vi "Begin.vi"(8 "error in":errorcluster) -> (0 "error out":errorcluster)   [LabVIEW 2016]
doc: "Called before other user functions, this VI is expected to open initial I/O refnums, load in file data, and do all program initialization. Notice that the <B>error out</B> terminal is simply used for data flow. Wiring it to other structures or subVIs ensures that this VI runs first."
uses:
  <vilib>/Rock Robotics/SystemInterfaces/DIO/FPGA_DIOPWMChannel.ctl
  <vilib>/Rock Robotics/WPI/SafetyOutput/WPI_SafetyOutputConfigMenu.ctl
  <vilib>/Rock Robotics/WPI/DriverStation/WPI_DriverStationRobotMode2.ctl
  <vilib>/Rock Robotics/WPI/Joystick/WPI_JoystickDeviceEnum.ctl
  <vilib>/Rock Robotics/WPI/Solenoid/WPI_SolenoidChannel.ctl
  <vilib>/Rock Robotics/SystemInterfaces/DIO/FPGA_DIOChannel.ctl
  <vilib>/Rock Robotics/WPI/Encoder/WPI_EncoderType.ctl
  <vilib>/Rock Robotics/WPI/RobotDrive/WPI_RobotDriveOpen2MotorWithTalon.vi
  Robot Global Data.vi
  <vilib>/Rock Robotics/Network Tables/SD Write String Array.vi
  <vilib>/Rock Robotics/WPI/Utilities/WPI_GetSetVariantRefNum.vi
  <vilib>/Rock Robotics/WPI/Solenoid/WPI_SolenoidOpenSingle.vi
  <vilib>/Rock Robotics/WPI/Counter/WPI_CounterDigitalInputToDigitalSource.vi
  <vilib>/Rock Robotics/WPI/MotorControl/WPI_MotorControlOpen VictorSP.vi
  <vilib>/Rock Robotics/WPI/Ultrasonic/WPI_SonarSRF04DigitalOpen.vi
  <vilib>/Rock Robotics/WPI/Ultrasonic/WPI_SonarSRF04DigitalRefNum Registry Set.vi
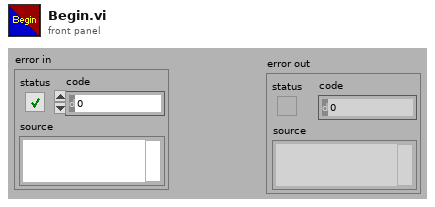
[diagram p1: front panel]
types:
  T1 = typedef "FPGA_DIOChannel.ctl" = enum8{"DIO 0", "DIO 1", "DIO 2", "DIO 3", "DIO 4", "DIO 5", "DIO 6", "DIO 7", "DIO 8", "DIO 9", "DIO MXP 0", "DIO MXP 1", "DIO MXP 2", "DIO MXP 3", "DIO MXP 4", "DIO MXP 5", "DIO MXP 6", "DIO MXP 7", "DIO MXP 8", "DIO MXP 9", "DIO MXP 10", "DIO MXP 11", "DIO MXP 12", "DIO MXP 13", "DIO MXP 14", "DIO MXP 15", "SPI Port CS1", "SPI Port CS2", "SPI Port CS3", "SPI Port MISO", "SPI Port MOSI", "Invalid"}
  T2 = typedef "FPGA_DIOPWMChannel.ctl" = enum8{"PWM 0", "PWM 1", "PWM 2", "PWM 3", "PWM 4", "PWM 5", "PWM 6", "PWM 7", "PWM 8", "PWM 9", "PWM MXP 0", "PWM MXP 1", "PWM MXP 2", "PWM MXP 3", "PWM MXP 4", "PWM MXP 5", "PWM MXP 6", "PWM MXP 7", "PWM MXP 8", "PWM MXP 9", "Invalid"}
  T3 = typedef "WPI_EncoderType.ctl" = enum16{"1x", "2x", "4x"}
  T4 = typedef "WPI_SolenoidChannel.ctl" = enum8{"Solenoid 0", "Solenoid 1", "Solenoid 2", "Solenoid 3", "Solenoid 4", "Solenoid 5", "Solenoid 6", "Solenoid 7", "Invalid"}
  T5 = typedef "WPI_JoystickDeviceEnum.ctl" = enum16{"USB 0", "USB 1", "USB 2", "USB 3", "USB 4", "USB 5"}
  T6 = typedef "WPI_DriverStationRobotMode2.ctl" = enum16{"Autonomous Disabled", "Autonomous Enabled", "Teleop Disabled", "Teleop Enabled", "Disconnected", "Finish", "Test Disabled", "Test Enabled", "Emergency Stopped"}
  T7 = typedef "WPI_SafetyOutputConfigMenu.ctl" = enum16{"Enable", "Disable"}
  T8 = typedef "WPI_DigitalInputDevRef.ctl" = cluster{"DevStatus":errorcluster, "DIO Channel":T1}
  T9 = typedef "FPGA_CounterEncoderSourceConvertionLVSourceType.ctl" = cluster{"DevStatus":errorcluster, "AnalogTriggerMode?":bool, "DigitalMode":cluster{"DIO Channel":T10}, "AnalogTriggerMode":cluster{"AnalogTriggerIndex":T11, "OutputType":T12}}
  T10 = typedef "FPGA_DIODigitalSourceChannel.ctl" = enum8{"DIO 0", "DIO 1", "DIO 2", "DIO 3", "DIO 4", "DIO 5", "DIO 6", "DIO 7", "DIO 8", "DIO 9", "DIO MXP 0", "DIO MXP 1", "DIO MXP 2", "DIO MXP 3", "DIO MXP 4", "DIO MXP 5", "DIO MXP 6", "DIO MXP 7", "DIO MXP 8", "DIO MXP 9", "DIO MXP 10", "DIO MXP 11", "DIO MXP 12", "DIO MXP 13", "DIO MXP 14", "DIO MXP 15", "Disabled"}
  T11 = typedef "FPGA_AnalogTriggerIndex.ctl" = enum8{"Trig 0", "Trig 1", "Trig 2", "Trig 3", "Trig 4", "Trig 5", "Trig 6", "Trig 7", "Invalid"}
  T12 = typedef "FPGA_AnalogTriggerOutType.ctl" = enum16{"InWindow", "TriggerState", "Rising", "Falling"}
  T13 = typedef "WPI_CompressorDevRef.ctl" = cluster{"DevStatus":errorcluster, "Pneumatics Control Module":u8}
  T14 = typedef "WPI_EncoderDevRef.ctl" = cluster{"DevStatus":errorcluster, "EncoderIndex":T15, "CounterIndex":T16, "DistancePerCount":dbl, "Decoding Type":T3}
  T15 = typedef "FPGA_EncoderIdx.ctl" = enum8{"Enc 0", "Enc 1", "Enc 2", "Enc 3", "Enc 4", "Enc 5", "Enc 6", "Enc 7", "Invalid"}
  T16 = typedef "FPGA_CounterCtrSystemIndex.ctl" = enum8{"Ctr 0", "Ctr 1", "Ctr 2", "Ctr 3", "Ctr 4", "Ctr 5", "Ctr 6", "Ctr 7", "Invalid"}
  T17 = typedef "WPI_SolenoidDevRef.ctl" = cluster{"DevStatus":errorcluster, "Pneumatics Control Module":u8, "Forward Solenoid Channel":T4, "Reverse Solenoid Channel":T4}
  T18 = typedef "WPI_JoystickDevRef.ctl" = cluster{"Device":T5}
  T19 = typedef "WPI_RobotDriveDevRef.ctl" = cluster{"DevStatus":errorcluster, "Motors[]":T20[], "Square Inputs":bool, "Max Output":dbl}
  T20 = typedef "WPI_MotorControlDeviceRef.ctl" = cluster{"DeviceStatus":errorcluster, "Type":T21, "PWM":cluster{"PWM Channel":T2, "DeadBand":T22}, "CAN":cluster{"Device Number":u8, "SetOutput VI Ref":variant, "GetOutput VI Ref":variant, "Enable VI Ref":variant, "Disable VI Ref":variant, "Data":variant}, "Invert":bool}
  T21 = typedef "WPI_MotorControlType.ctl" = enum16{"PWM", "CAN"}
  T22 = typedef "WPI_PWMDeadband.ctl" = cluster{"Name":string, "maxPositivePwm":i32, "minPositivePwm":i32, "centerPwm":i32, "maxNegativePwm":i32, "minNegativePwm":i32, "angularRange":u16}
  T23 = typedef "WPI_UltrasonicDeviceRef.ctl" = cluster{"DevStatus":errorcluster, "Ping Channel":T1, "Echo Channel":T1, "CntIndex":T16}
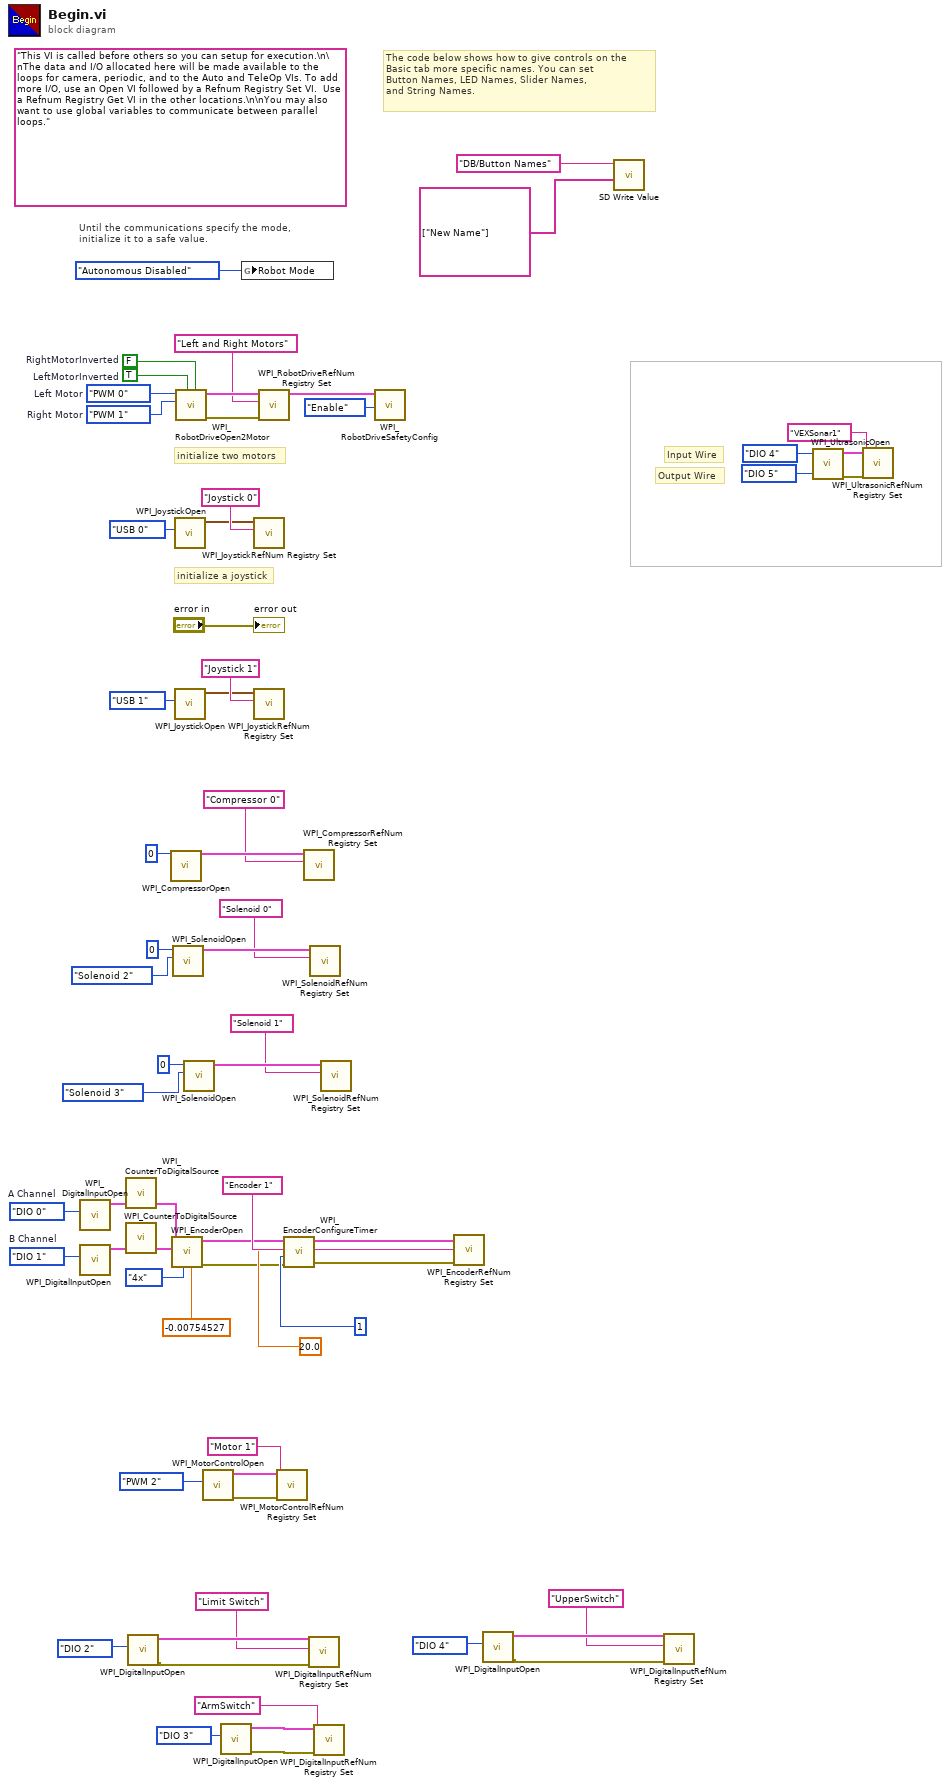
[diagram p0: block diagram]
diagram:
  w36 = FPGA_DIOChannel."DIO 1"  # B Channel
  w35 = FPGA_DIOChannel."DIO 0"  # A Channel
  (unwired) "This VI is called before others so you can setup for execution.\n\nThe data and I/O allocated here will be made available to the loops for camera, periodic, and to the Auto and TeleOp VIs. To add more I/O, use an Open VI followed by a Refnum Registry Set VI.  Use a Refnum Registry Get VI in the other locations.\n\nYou may also want to use global variables to communicate between parallel loops."
  w60 = FPGA_DIOPWMChannel."PWM 1"  # Right Motor
  w61 = FPGA_DIOPWMChannel."PWM 0"  # Left Motor
  w65 = TRUE  # LeftMotorInverted
  w66 = FALSE  # RightMotorInverted
  # "Output Wire"
  # "Input Wire"
  # "The code below shows how to give controls on the\nBasic tab more specific names. You can set\nButton Names, LED Names, Slider Names,\nand String Names."
  # "initialize a joystick"
  # "Until the communications specify the mode,\ninitialize it to a safe value."
  # "initialize two motors"
  n1 = call <vilib>:"WPI_DigitalInputOpen.vi"("DIO Channel"=w35) -> ("DigitalInputDevRef"=w32:T8)  [unwired: 1 in, 9 out]
  n2 = call <vilib>:"WPI_DigitalInputOpen.vi"("DIO Channel"=w36) -> ("DigitalInputDevRef"=w33:T8)  [unwired: 1 in, 9 out]
  n3 = call-poly <vilib>:"WPI_CounterToDigitalSource.vi"("DigitalInputDevRef"=w32) -> ("Digital Source"=w31:T9)  [unwired: 6 out]
  n4 = call-poly <vilib>:"WPI_CounterToDigitalSource.vi"("DigitalInputDevRef"=w33) -> ("Digital Source"=w34:T9)  [unwired: 6 out]
  n5 = call <vilib>:"WPI_DigitalInputOpen.vi"("DIO Channel"=FPGA_DIOChannel."DIO 2") -> ("error out"=w21:errorcluster, "DigitalInputDevRef"=w26:T8)  [unwired: 9 in]
  n6 = call <vilib>:"WPI_CompressorOpen.vi"("Pneumatics Control Module (0)"=u8 0) -> ("CompressorDevRef"=w46:T13)  [unwired: 13 in, 1 out]
  n7 = call <vilib>:"WPI_EncoderOpen.vi"("DistancePerCount"=-0.00754527, "Decoding Type"=WPI_EncoderType."4x", "BSource"=w34, "ASource"=w31) -> ("error out"=w20:errorcluster, "EncoderDevRef"=w29:T14)  [unwired: 4 in, 2 out]
  n8 = call-poly <vilib>:"WPI_SolenoidOpen.vi"("Solenoid Channel"=WPI_SolenoidChannel."Solenoid 2" ("Forward Solenoid Channel"), "Pneumatics Control Module (0)"=u8 0) -> ("SolenoidDevRef"=w44:T17)  [unwired: 8 in, 1 out]
  n9 = call <vilib>:"WPI_JoystickOpen.vi"("JoystickDevice"=WPI_JoystickDeviceEnum."USB 0") -> ("JoystickDevRef"=w55:T18)  [unwired: 10 in]
  n10 = call <vilib>:"WPI_JoystickOpen.vi"("JoystickDevice"=WPI_JoystickDeviceEnum."USB 1") -> ("JoystickDevRef"=w49:T18)  [unwired: 10 in]
  n11 = call-poly <vilib>:"WPI_RobotDriveOpen2Motor.vi"("Right Motor Inverted"=w66, "Left Motor Inverted"=w65, "Right Motor"=w60, "Left Motor"=w61) -> ("error out"=w62:errorcluster, "RobotDriveDevRef"=w64:T19)  [unwired: 1 in, 5 out]
  n12 = call-poly <vilib>:"WPI_SolenoidOpen.vi"("Solenoid Channel"=WPI_SolenoidChannel."Solenoid 3" ("Forward Solenoid Channel"), "Pneumatics Control Module (0)"=u8 0) -> ("SolenoidDevRef"=w40:T17)  [unwired: 8 in, 1 out]
  n13 = call-poly <vilib>:"WPI_MotorControlOpen.vi"("PWM Channel"=FPGA_DIOPWMChannel."PWM 2") -> ("error out"=w17:errorcluster, "MotorControlDeviceRef"=w16:T20)  [unwired: 9 in]
  n14 = call <vilib>:"WPI_DigitalInputOpen.vi"("DIO Channel"=FPGA_DIOChannel."DIO 3") -> ("error out"=w13:errorcluster, "DigitalInputDevRef"=w12:T8)  [unwired: 9 in]
  n15 = global write "Robot Global Data.vi" "Robot Mode"(WPI_DriverStationRobotMode2."Autonomous Disabled" ("Robot Mode")) -> ()
  n16 = call <vilib>:"WPI_JoystickRefNum Registry Set.vi"("refnum name"="Joystick 0", "JoystickDevRef"=w55) -> ()  [unwired: 8 in, 2 out]
  n17 = call <vilib>:"WPI_JoystickRefNum Registry Set.vi"("refnum name"="Joystick 1", "JoystickDevRef"=w49) -> ()  [unwired: 8 in, 2 out]
  n18 = call <vilib>:"WPI_RobotDriveRefNum Registry Set.vi"("error in (no error)"=w62, "refnum name"="Left and Right Motors", "RobotDriveDevRef"=w64) -> ("RobotDriveDevRef"=w59:T19)  [unwired: 1 in, 7 out]
  n19 = call <vilib>:"WPI_MotorControlRefNum Registry Set.vi"("error in (no error)"=w17, "refnum name"="Motor 1", "MotorControlDevRef"=w16) -> ()  [unwired: 7 in, 2 out]
  n20 = call <vilib>:"WPI_EncoderConfigureTimer.vi"("error in (no error)"=w20, "Number Samples to Average"=u8 1, "Minimum Rate"=20.0, "EncoderDevRef"=w29) -> ("error out"=w19:errorcluster, "EncoderDevRef"=w28:T14)  [unwired: 6 in]
  n21 = call <vilib>:"WPI_CompressorRefNum Registry Set.vi"("refnum name"="Compressor 0", "CompressorDevRef"=w46) -> ()  [unwired: 8 in, 2 out]
  n22 = call <vilib>:"WPI_DigitalInputRefNum Registry Set.vi"("error in (no error)"=w21, "refnum name"="Limit Switch", "DigitalInputDevRef"=w26) -> ()  [unwired: 7 in, 2 out]
  n23 = call <vilib>:"WPI_SolenoidRefNum Registry Set.vi"("refnum name"="Solenoid 0", "SolenoidDevRef"=w44) -> ()  [unwired: 8 in, 2 out]
  n24 = call <vilib>:"WPI_DigitalInputRefNum Registry Set.vi"("error in (no error)"=w13, "refnum name"="ArmSwitch", "DigitalInputDevRef"=w12) -> ()  [unwired: 7 in, 2 out]
  n25 = call <vilib>:"WPI_SolenoidRefNum Registry Set.vi"("refnum name"="Solenoid 1", "SolenoidDevRef"=w40) -> ()  [unwired: 8 in, 2 out]
  n26 = call <vilib>:"WPI_RobotDriveSafetyConfig.vi"("mode"=WPI_SafetyOutputConfigMenu."Enable", "RobotDriveDevRef"=w59) -> ()  [unwired: 8 in, 2 out]
  n27 = call <vilib>:"WPI_EncoderRefNum Registry Set.vi"("error in (no error)"=w19, "refnum name"="Encoder 1", "EncoderDevRef"=w28) -> ()  [unwired: 7 in, 2 out]
  n28 = call <vilib>:"WPI_DigitalInputOpen.vi"("DIO Channel"=FPGA_DIOChannel."DIO 4") -> ("error out"=w6:errorcluster, "DigitalInputDevRef"=w8:T8)  [unwired: 9 in]
  n29 = call-poly <vilib>:"SD Write Value.vi"("String Array"=string[] ["New Name"], "Name"="DB/Button Names") -> ()  [unwired: 8 in, 2 out]
  n30 = call <vilib>:"WPI_DigitalInputRefNum Registry Set.vi"("error in (no error)"=w6, "refnum name"="UpperSwitch", "DigitalInputDevRef"=w8) -> ()  [unwired: 7 in, 2 out]
  n31 = call-poly <vilib>:"WPI_UltrasonicOpen.vi"("Echo DIO Channel"=FPGA_DIOChannel."DIO 5", "Ping DIO Channel"=FPGA_DIOChannel."DIO 4") -> ("error out"=w5:errorcluster, "SonarSRF04DevRef"=w4:T23)  [unwired: 8 in]
  n32 = call-poly <vilib>:"WPI_UltrasonicRefNum Registry Set.vi"("error in (no error)"=w5, "refnum name"="VEXSonar1", "SonarSRF04DevRef"=w4) -> ()  [unwired: 7 in, 2 out]
  "error out" <- "error in"
